vi "Configure Timestamp Rate.vi"(8 "error in (no error)":errorcluster, 10 "Rate (1E+6)":dbl=1000000.0, 11 "VISA resource name":refnum<visa-resource-name>) -> (0 "error out":errorcluster, 3 "VISA resource name out":refnum<visa-resource-name>)   [LabVIEW 2021, in "Agilent 532XX Series.lvlib"]
doc: "Selects the nominal rate at which timestamp data is produced. The actual rate will depend on the input frequency.\n\n<B>Note:</B> This VI only applies to the Agilent 53230A."
uses:
  <instrlib>/Agilent 532XX Series/Agilent 532XX Series.lvlib
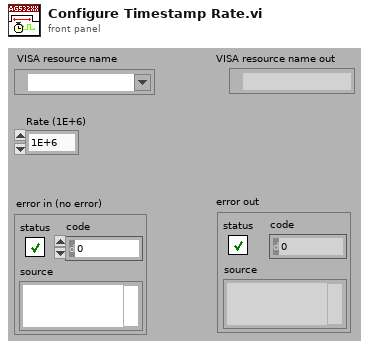
[diagram p1: front panel]
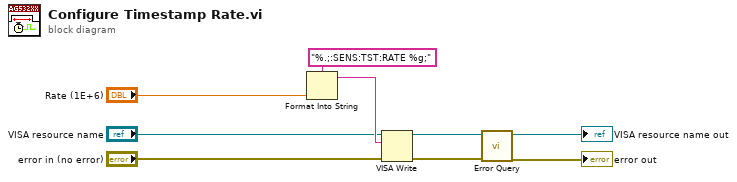
[diagram p0: block diagram]
diagram:
  n1 = Format Into String(format string="%.;:SENS:TST:RATE %g;", "Rate (1E+6)") -> (resulting string=w7:string)  [unwired: 2 in, 1 out]
  n2 = VISA Write(VISA resource name="VISA resource name", write buffer=w7, error in (no error)="error in (no error)") -> (VISA resource name out=w4:refnum<visa-resource-name>, error out=w3:errorcluster)  [unwired: 1 out]
  n3 = call <instrlib>:"Error Query.vi"("error in (no error)"=w3, "VISA resource name"=w4) -> ("error out"=→"error out":errorcluster, "VISA resource name out"=→"VISA resource name out":refnum<visa-resource-name>)  [unwired: 8 out]
